vi "Configure Stop Trigger [SPT].vi"(7 "Trigger Slope (Positive)":i32(ring) caption="trigger slope (Positive)" items=["Positive", "Negative", "Either"], 8 "error in (no error)":errorcluster, 9 "Trigger Source (None)":string(combo) caption="trigger source (None)", 10 "Channel Name (\"\")":string="CHANNEL1" caption="channel name (\"CHANNEL1\")", 11 "CS++Fgen in":refnum<class "CS++Fgen.lvclass">) -> (0 "error out":errorcluster, 3 "Fgen out":refnum<class "CS++Fgen.lvclass">)   [LabVIEW 2015, in "CS++Fgen.lvlib" / "CS++Fgen.lvclass"]
doc: "This VI configures the properties that control the function generator's stop trigger. These properties are the stop trigger source and slope.\n\nA stop trigger terminates any generation and has the same effect as calling the IviFgen Abort Generation VI.\n\nNote:\n\n(1) This VI is part of the IviFgenStopTrigger [SPT] extension group."
uses:
  CS++Fgen.lvclass
  CSPP_Core/Classes/CS++ProcessVariables/ProcessVariable/PV.lvclass
  PV-Enum-n.ctl
  CSPP_Core/Classes/CS++ProcessVariables/ProcessVariable/PV.lvclass/PV.ctl
  CS++Fgen.lvclass/CS++Fgen.ctl
  CSPP_Core/Classes/CS++ProcessVariables/ProcessVariable/Write Data.vi
  CSPP_Core/Classes/CS++ProcessVariables/ProcessVariable/Write Timestamp.vi
  CSPP_Core/Classes/CS++ProcessVariables/ProcessVariable/Write Quality.vi
  CSPP_Core/Classes/CS++ProcessVariables/ProcessVariable/Write status.vi
  CSPP_Core/Classes/CS++ProcessVariables/PVConnection/PVConnection.lvclass
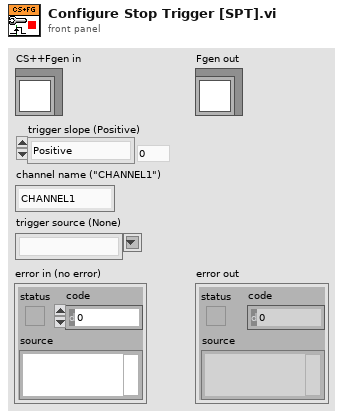
[diagram p1: front panel]
types:
  T1 = typedef "CS++Fgen.lvlib/CS++Fgen.lvclass/PV-Enum-n.ctl" = enum16{"Amplitude", "Arb-Frequency", "DCOffset", "Frequency", "OutputImpedance", "StartPhase", "AdvancedTriggerSlope", "AM-Source", "BurstCount", "FM-Source", "OperationMode", "ResumeTriggerSlope", "StartTriggerSlope", "StopTriggerSlope", "Waveform", "TriggerSource", "AM-Enabled", "ChannelEnabled", "FM-Enabled", "AdvancedTriggerSource", "ResumeTriggerSource", "StartTriggerSource", "StopTriggerSource"}
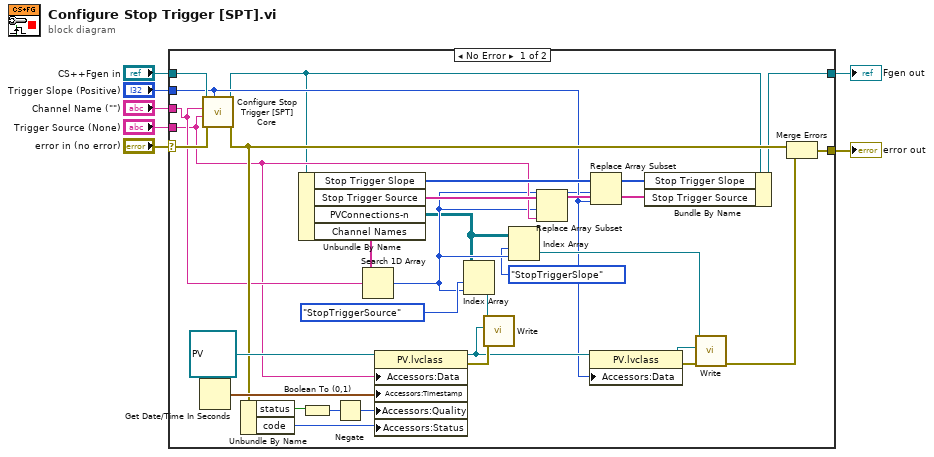
[diagram p0: block diagram]
diagram:
  n1 = case shown="No Error" "error in (no error)" {
    selector: "error in (no error)" -> [w37 w40]
    tunnel: [w12 w40] -> w6
    tunnel: [w13 w39] -> w4
    tunnel: "CS++Fgen in" -> [w38 w39]
    tunnel: "Trigger Slope (Positive)" -> [w15 _]
    tunnel: "Channel Name (\"\")" -> [w17 _]
    tunnel: "Trigger Source (None)" -> [w16 _]
    frame No Error {
      n2 = Get Date/Time In Seconds() -> (seconds since 1Jan1904=w36:timestamp)
      n3 = call-dynamic "Configure Stop Trigger [SPT] Core.vi"("Trigger Slope (Positive)"=w15, "error in (no error)"=w37, "Trigger Source (None)"=w16, "Channel Name (\"\")"=w17, "CS++Fgen in"=w38) -> ("error out"=w18:errorcluster, "Fgen out"=w14:refnum<class "CS++Fgen.lvclass">)  [unwired: 5 in]
      n4 = Unbundle By Name(w18) -> ("status"=w31:bool, "code"=w29:i32)
      n5 = Unbundle By Name(w14) -> ("Stop Trigger Slope"=w25:i32[], "Stop Trigger Source"=w27:string[], "PVConnections-n"=w8:refnum<class "PVConnection.lvclass">[][], "Channel Names"=w33:string[])
      n6 = Boolean To (0,1)(Boolean=w31) -> (0, 1=w30:i16)
      n7 = Negate(x=w30) -> (-x=w28:i16)
      n8 = Search 1D Array(1D array=w33, element=w17) -> (index of element=w10:i32)  [unwired: 1 in]
      n9 = property class="PV.lvclass"(reference=refnum<class "PV.lvclass"> refnum ("PV"), "Accessors:Data"=w16, "Accessors:Timestamp"=w36, "Accessors:Quality"=w28, "Accessors:Status"=w29) -> (reference out=w21:refnum<class "PV.lvclass">, error out=w34:errorcluster)  [unwired: 1 in]
      n10 = Index Array(array=w8, index (row)=PV-Enum-n."StopTriggerSource" ("PV-Enum-n"), index (col)=w10) -> (element=w32:refnum<class "PVConnection.lvclass">)
      n11 = call "Write.vi"("error in (no error)"=w34, "PV"=w21, "PVConnection in"=w32) -> ()  [unwired: 7 in, 2 out]
      n12 = Index Array(array=w8, index (row)=PV-Enum-n."StopTriggerSlope" ("PV-Enum-n"), index (col)=w10) -> (element=w20:refnum<class "PVConnection.lvclass">)
      n13 = Replace Array Subset(array=w27, new element=w16, index=w10) -> (w26:string[])
      n14 = property class="PV.lvclass"(reference=w21, "Accessors:Data"=w15) -> (reference out=w23:refnum<class "PV.lvclass">, error out=w22:errorcluster)  [unwired: 1 in]
      n15 = Replace Array Subset(array=w25, new element=w15, index=w10) -> (w24:i32[])
      n16 = Bundle By Name(cluster=w14, "Stop Trigger Slope"=w24, "Stop Trigger Source"=w26) -> (w13:refnum<class "CS++Fgen.lvclass">)
      n17 = call "Write.vi"("error in (no error)"=w22, "PV"=w23, "PVConnection in"=w20) -> ("error out"=w19:errorcluster)  [unwired: 7 in, 1 out]
      n18 = Merge Errors(w18, w19) -> (w12:errorcluster)
    }
    frame Error {
    }
  }
  "error out" <- w6
  "Fgen out" <- w4
